vi "ezAFM Practice 1.8.vi"() -> ()   [LabVIEW 2015]
uses:
  <vilib>/userdefined/High Color/IMAQdx.ctl
  D:/LabVIEW for ezAFM/LV-PGC 2019-05a/Special Equipment/ezAFM/NMI Integration Code/ezCommander.dll
  LabVIEW for ezAFM/LV-PGC 2019-05a/Special Equipment/ezAFM/NMI Integration Code/ezCommander.dll
  LabVIEW for ezAFM/LV-PGC 2019-05a/Universal vi's/Global Variables/Globals-EasyAFM.vi
  Helper VI's/Globals.vi
  <vilib>/vision/driver/NI_Vision_Acquisition_Software.lvlib
panel:
  out "Scan Spot Coordinates":dbl[](array[numeric])
  out "Name":string
  out "Sequence Index":dbl
  out "Direction":dbl
  out "Searching":bool
  out "Crosshair Found?":bool
  in  "Search":bool
  out "Total Steps":dbl
  out "Current Steps":dbl
  in  "Camera":enum32{"ezAFM Camera"}(tab)
  out "ezAFM Camera":T1(plugin-control)
  in  "Connection to Scan":string
  in  "Enable Automatic \nRepositioning":bool
  out "Imaging Status":string
  out "Automated Imaging":bool
  in  "Main Menu":T2(tab)
  in  "Navigation Buttons":T3
  in  "Motor Speed":u16(ring)=30000 items=["SLOW"=3300, "MEDIUM"=30000, "FAST"=65000]
  in  "Target Crosshair":string(combo)="00 | 01"
  in  "Current Crosshair":string(combo)="00 | 01"
  in  "MOVE2CROSSHAIR":bool
  in  "THETA":bool
  in  "Angle":dbl
  in  "Step Size":dbl
  in  "Scan Spot":string(combo)
  in  "MOVE2SCANSPOT":bool
  in  "RETRACT":bool
  in  "APPROACH":bool
  in  "SEARCH":bool
  in  "SCAN":bool
  in  "Image Resolution":u16(ring)=256 items=["128"=128, "256"=256, "512"=512, "1024"=1024]
  out "Sequence":string[](array[string])
  out "Connections":string[](array[string])
  in  "Initialize Automated Imaging":bool
  in  "SELECT CONNECTIONS":bool
  in  "ezAFM Default File Path":path=path "D:/ezAFM/Scanned Images"
  in  "Saved Images File Path":path=path "D:/ezAFM/Scanned Images"
  in  "Wafer Type":string(combo)
  in  "Die":string(combo)
  in  "Indicators":enum32{"Indicators"}(tab)
  out "XYZ Motor Position":dbl[](array[numeric]) format="%#_4f"
  out "ezAFM Status":dbl
  out "Approaching":bool
  out "ezAFM Connected":bool
  out "Retracting":bool
  out "Scanning":bool
  out "Tip Approached?":bool
  in  "RESET":bool
  out "XY Position":dbl[](array[numeric])
  in  "QUIT":bool
  # "Use Arrow Keys to manually\nmove the XY Motor"
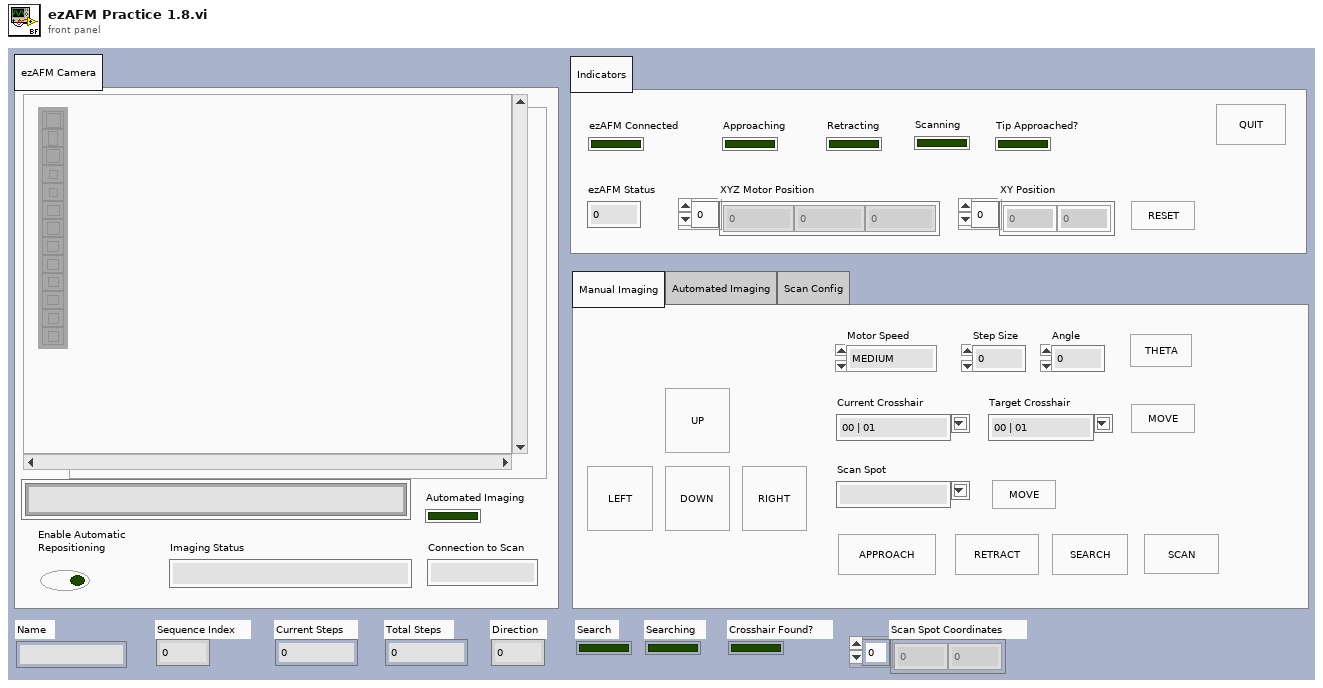
[diagram p1: front panel]
types:
  T1 = typedef "IMAQ Image.ctl" = refnum<image>
  T2 = enum32{"Manual Imaging", "Automated Imaging", "Scan Config"}
  T3 = cluster{"UP":bool, "DOWN":bool, "LEFT":bool, "RIGHT":bool}
  T4 = typedef "IMAQdx.ctl" = refnum<k21>
  T5 = typedef "Image Type" = u32
  T6 = typedef "eventvkey.ctl" = enum16{"ASCII", "Enter", "Return", "Shift", "Ctrl", "Alt", "Cmd", "Opt", "Caps", "NumLock", "Clear", "Break", "Up", "Down", "Left", "Right", "Insert", "Delete", "Home", "End", "PageUp", "PageDown", "Escape", "Help", "Pause", "ScrollLock", "F1", "F2", "F3", "F4", "F5", "F6", "F7", "F8", "F9", "F10", "F11", "F12", "F13", "F14", "F15", "F16", "F17", "F18", "F19", "F20", "F21", "F22", "F23", "F24", "Play", "VolumeUp", "VolumeDown", "Mute", "Two Byte Char"}
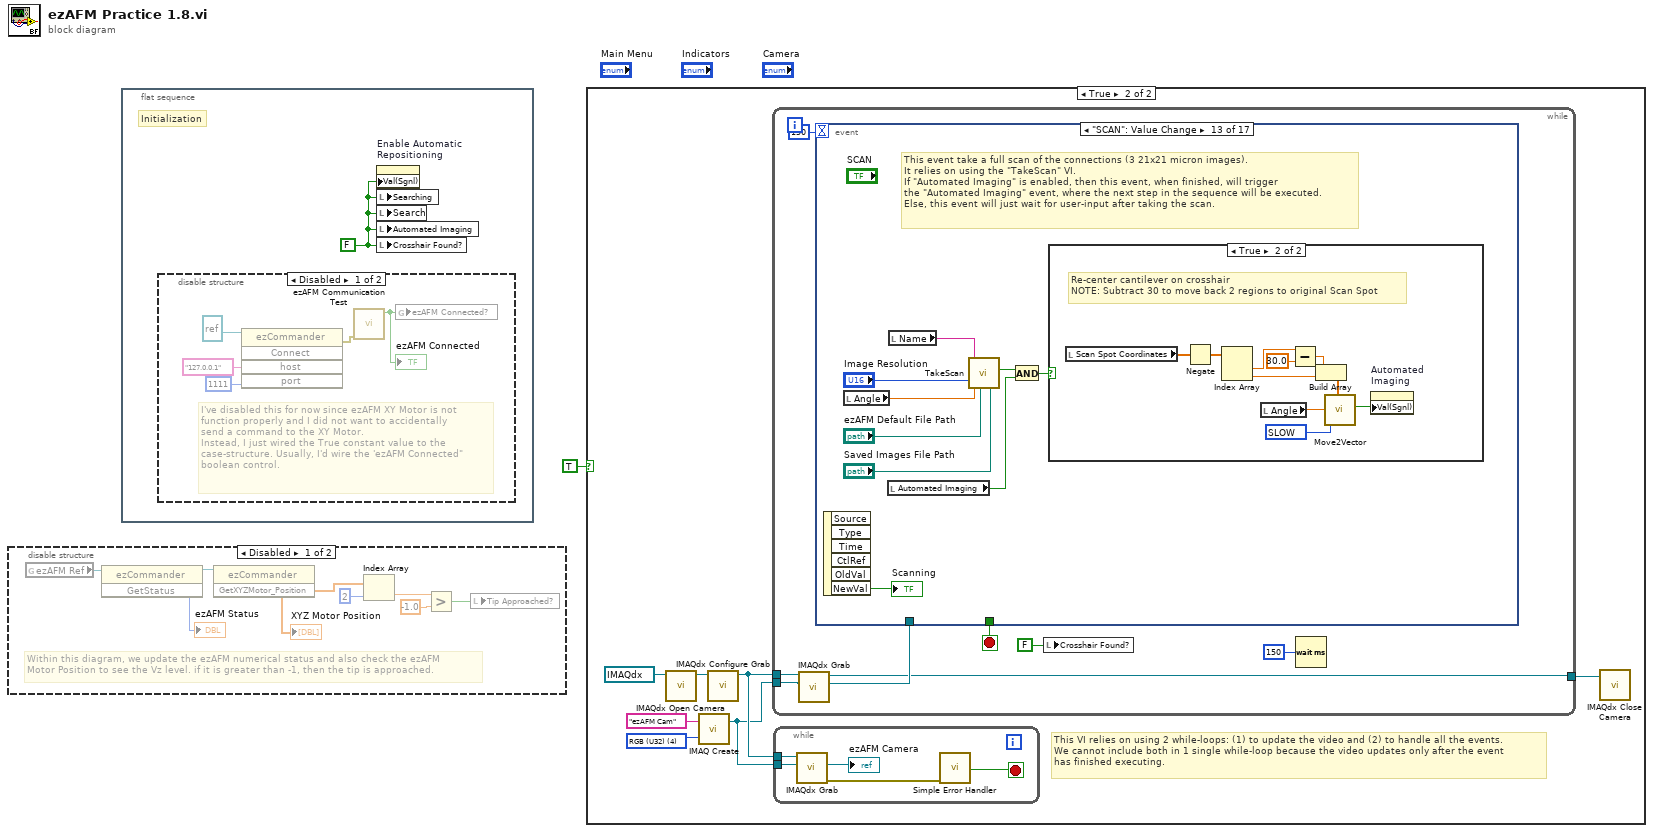
[diagram p0: block diagram]
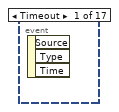
[diagram p5: hidden frame]
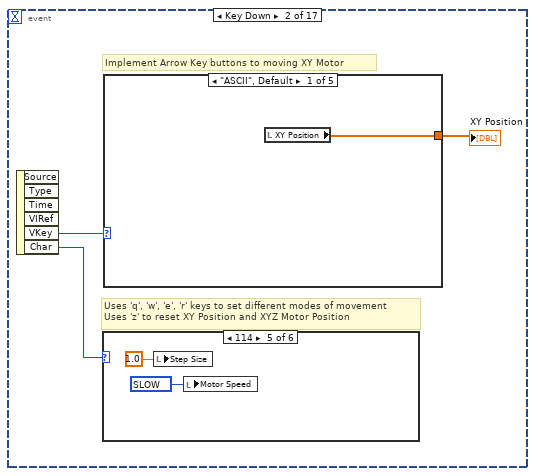
[diagram p6: hidden frame]
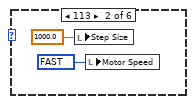
[diagram p8: hidden frame]
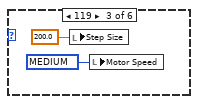
[diagram p9: hidden frame]
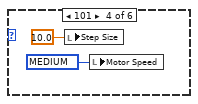
[diagram p10: hidden frame]
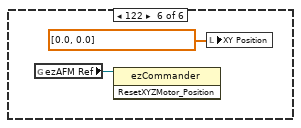
[diagram p11: hidden frame]
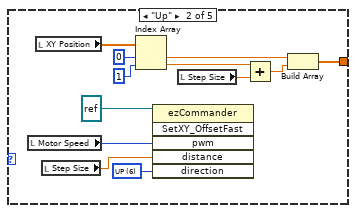
[diagram p12: hidden frame]
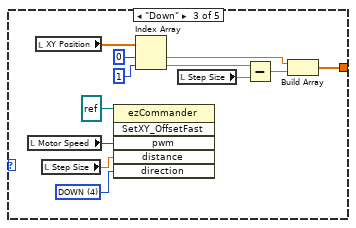
[diagram p13: hidden frame]
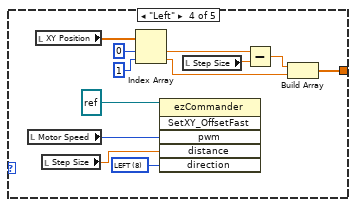
[diagram p14: hidden frame]
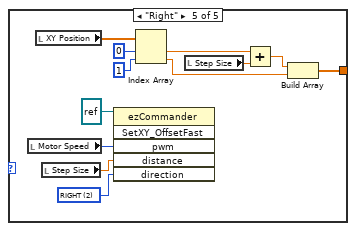
[diagram p15: hidden frame]
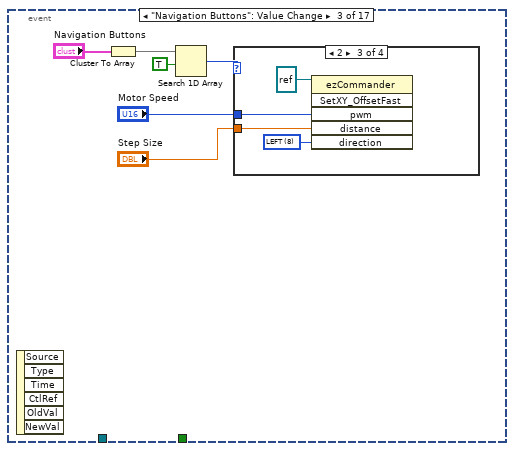
[diagram p16: hidden frame]
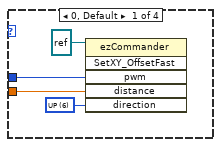
[diagram p17: hidden frame]
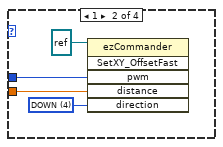
[diagram p18: hidden frame]
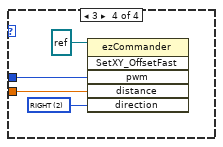
[diagram p19: hidden frame]
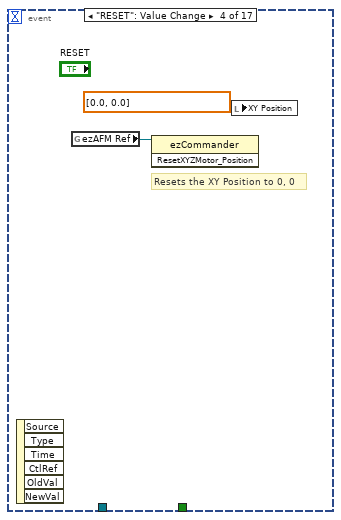
[diagram p20: hidden frame]
diagram:
  n1 = disable-structure shown="Disabled" {
    frame Disabled {
      # "Within this diagram, we update the ezAFM numerical status and also check the ezAFM\nMotor Position to see the Vz level. if it is greater than -1, then the tip is approached."
      n2 = global read "Globals-EasyAFM.vi" "ezAFM Ref"() -> (w7:refnum<k24>)
      n3 = invoke class="ezCommander" method="GetStatus"(reference=w7) -> (reference out=w5:refnum<k24>, "GetStatus"=→"ezAFM Status":i32)  [unwired: 2 in, 1 out]
      n4 = invoke class="ezCommander" method="GetXYZMotor_Position"(reference=w5) -> ("GetXYZMotor_Position"=w9:dbl[])  [unwired: 2 in, 2 out]
      "XYZ Motor Position" <- w9
      n5 = Index Array(array=w9, index=2) -> (element=w4:dbl)
      n6 = Greater?(x=w4, y=-1.0) -> (0:w8:bool)
      n7 = local write "Tip Approached?"(w8) -> ()
    }
    frame Enabled {
    }
  }
  n8 = flat-sequence {
    frame #0 {
      w10 = FALSE ("Automated Imaging")
      # "Initialization"
      n9 = disable-structure shown="Disabled" {
        frame Disabled {
          # "I've disabled this for now since ezAFM XY Motor is not \nfunction properly and I did not want to accidentally\nsend a command to the XY Motor. \nInstead, I just wired the True constant value to the \ncase-structure. Usually, I'd wire the 'ezAFM Connected\"\nboolean control."
          n10 = invoke class="ezCommander" method="Connect"(reference=refnum<k24> refnum ("ezAFM Ref"), "host"="127.0.0.1", "port"=1111) -> (error out=w14:errorcluster)  [unwired: 2 in, 4 out]
          n11 = call "ezAFM Communication Test.vi"("error in"=w14) -> ("ezAFM COM status"=w11:bool)  [unwired: 3 in, 3 out]
          "ezAFM Connected" <- w11
          n12 = global write "Globals.vi" "ezAFM Connected?"(w11) -> ()
        }
        frame Enabled {
        }
      }
      n13 = property on="Enable Automatic \nRepositioning" class="Bool (strict)"("Val(Sgnl)"=w10) -> ()  [unwired: 2 in, 2 out]
      n14 = local write "Searching"(w10) -> ()
      n15 = local write "Search"(w10) -> ()
      n16 = local write "Automated Imaging"(w10) -> ()
      n17 = local write "Crosshair Found?"(w10) -> ()
    }
  }
  n18 = case shown="True" TRUE {
    frame False {
    }
    frame True {
      w19 = T5 4 items=["Grayscale (U8)", "Grayscale (I16)", "Grayscale (SGL)", "Complex (CSG)", "RGB (U32)", "HSL (U32)", "RGB (U64)", "Grayscale (U16)"] ("Image Type")
      # "This VI relies on using 2 while-loops: (1) to update the video and (2) to handle all the events.\nWe cannot include both in 1 single while-loop because the video updates only after the event\nhas finished executing."
      n19 = call <vilib>:"IMAQdx Open Camera.vi"("Session In"=T4 "cam5") -> ("Session Out"=w20:T4)  [unwired: 9 in, 1 out]
      n20 = call "IMAQ Create"("Image Name"="ezAFM Cam", "Image Type"=w19) -> ("New Image"=w17:T1)  [unwired: 3 in, 1 out]
      n21 = call <vilib>:"IMAQdx Configure Grab.vi"("Session In"=w20) -> ("Session Out"=w18:T4)  [unwired: 9 in, 1 out]
      n22 = while {
        tunnel: w18 -> [w33]
        tunnel: w17 -> [w32]
        tunnel: [w30] -> w16
        stop <- w29 stop-if-true
        n23 = call <vilib>:"IMAQdx Grab.vi"("Image In"=w32, "Session In"=w33) -> ("Image Out"=w31:T1, "Session Out"=w30:T4)  [unwired: 2 in, 6 out]
        n24 = event shown="[12] \"SCAN\": Value Change" {
          selector: _ -> [_ _ _ _ _ _ _ _ _ _ _ _ _ _ _ _ _]
          dyn-events: _ -> [_ _ _ _ _ _ _ _ _ _ _ _ _ _ _ _ _]
          timeout: 150 -> [_ _ _ _ _ _ _ _ _ _ _ _ _ _ _ _ _]
          tunnel: [_ _ _ _ _ _ _ _ _ _ _ _ _ _ _ _ "QUIT"] -> w29
          tunnel: w31 -> [_ _ _ _ _ _ _ _ _ _ _ _ _ _ w273 _ _]
          event Timeout {
            n25 = event-data() -> ()  [unwired: 1 in, 3 out]
          }
          event Key Down {
            # "Uses 'q', 'w', 'e', 'r' keys to set different modes of movement\nUses 'z' to reset XY Position and XYZ Motor Position"
            # "Implement Arrow Key buttons to moving XY Motor"
            n26 = event-data() -> ("VKey"=w36:T6, "Char"=w37:i16)  [unwired: 1 in, 4 out]
            n27 = case shown="114" w37 {
              frame 0, Default {
              }
              frame 113 {
                w39 = u16 65000 items=["SLOW"=3300, "MEDIUM"=30000, "FAST"=65000] ("Motor Speed")
                n28 = local write "Step Size"(1000.0 ("Step Size")) -> ()
                n29 = local write "Motor Speed"(w39) -> ()
              }
              frame 119 {
                w41 = u16 30000 items=["SLOW"=3300, "MEDIUM"=30000, "FAST"=65000] ("Motor Speed")
                n30 = local write "Step Size"(200.0 ("Step Size")) -> ()
                n31 = local write "Motor Speed"(w41) -> ()
              }
              frame 101 {
                w43 = u16 30000 items=["SLOW"=3300, "MEDIUM"=30000, "FAST"=65000] ("Motor Speed")
                n32 = local write "Step Size"(10.0 ("Step Size")) -> ()
                n33 = local write "Motor Speed"(w43) -> ()
              }
              frame 114 {
                w45 = u16 3300 items=["SLOW"=3300, "MEDIUM"=30000, "FAST"=65000] ("Motor Speed")
                n34 = local write "Step Size"(1.0 ("Step Size")) -> ()
                n35 = local write "Motor Speed"(w45) -> ()
              }
              frame 122 {
                n36 = global read "Globals-EasyAFM.vi" "ezAFM Ref"() -> (w47:refnum<k24>)
                n37 = invoke class="ezCommander" method="ResetXYZMotor_Position"(reference=w47) -> ()  [unwired: 2 in, 3 out]
                n38 = local write "XY Position"(dbl[] [0.0, 0.0] ("XY Position")) -> ()
              }
            }
            n39 = case shown="\"ASCII\", Default" w36 {
              tunnel: [w49 w51 w62 w74 w86] -> w38
              frame "ASCII", Default {
                n40 = local read "XY Position"() -> (w49:dbl[])
              }
              frame "Up" {
                w60 = u16 6 items=["UP"=6, "DOWN"=4, "LEFT"=8, "RIGHT"=2]
                n41 = local read "Motor Speed"() -> (w59:u16)
                n42 = local read "XY Position"() -> (w57:dbl[])
                n43 = local read "Step Size"() -> (w58:dbl)
                n44 = Index Array(array=w57, index #1=0 ("index"), index #2=1 ("index")) -> (element #1=w53:dbl, element #2=w50:dbl)
                n45 = invoke class="ezCommander" method="SetXY_OffsetFast"(reference=refnum<k24> refnum ("ezAFM Ref"), "pwm"=w59, "distance"=w58, "direction"=w60) -> ()  [unwired: 2 in, 6 out]
                n46 = local read "Step Size"() -> (w54:dbl)
                n47 = Add(x=w50, y=w54) -> (x+y=w52:dbl)
                n48 = Build Array(w53, w52) -> (w51:dbl[])
              }
              frame "Down" {
                w70 = u16 4 items=["UP"=6, "DOWN"=4, "LEFT"=8, "RIGHT"=2]
                n49 = local read "Motor Speed"() -> (w72:u16)
                n50 = local read "XY Position"() -> (w64:dbl[])
                n51 = local read "Step Size"() -> (w71:dbl)
                n52 = invoke class="ezCommander" method="SetXY_OffsetFast"(reference=refnum<k24> refnum ("ezAFM Ref"), "pwm"=w72, "distance"=w71, "direction"=w70) -> ()  [unwired: 2 in, 6 out]
                n53 = Index Array(array=w64, index #1=0 ("index"), index #2=1 ("index")) -> (element #1=w66:dbl, element #2=w67:dbl)
                n54 = local read "Step Size"() -> (w63:dbl)
                n55 = Subtract(x=w67, y=w63) -> (x-y=w65:dbl)
                n56 = Build Array(w66, w65) -> (w62:dbl[])
              }
              frame "Left" {
                w84 = u16 8 items=["UP"=6, "DOWN"=4, "LEFT"=8, "RIGHT"=2]
                n57 = local read "Motor Speed"() -> (w82:u16)
                n58 = local read "XY Position"() -> (w78:dbl[])
                n59 = local read "Step Size"() -> (w83:dbl)
                n60 = Index Array(array=w78, index #1=0 ("index"), index #2=1 ("index")) -> (element #1=w77:dbl, element #2=w75:dbl)
                n61 = invoke class="ezCommander" method="SetXY_OffsetFast"(reference=refnum<k24> refnum ("ezAFM Ref"), "pwm"=w82, "distance"=w83, "direction"=w84) -> ()  [unwired: 2 in, 6 out]
                n62 = local read "Step Size"() -> (w79:dbl)
                n63 = Subtract(x=w77, y=w79) -> (x-y=w76:dbl)
                n64 = Build Array(w76, w75) -> (w74:dbl[])
              }
              frame "Right" {
                w96 = u16 2 items=["UP"=6, "DOWN"=4, "LEFT"=8, "RIGHT"=2]
                n65 = local read "Motor Speed"() -> (w95:u16)
                n66 = local read "XY Position"() -> (w91:dbl[])
                n67 = local read "Step Size"() -> (w94:dbl)
                n68 = invoke class="ezCommander" method="SetXY_OffsetFast"(reference=refnum<k24> refnum ("ezAFM Ref"), "pwm"=w95, "distance"=w94, "direction"=w96) -> ()  [unwired: 2 in, 6 out]
                n69 = Index Array(array=w91, index #1=0 ("index"), index #2=1 ("index")) -> (element #1=w89:dbl, element #2=w87:dbl)
                n70 = local read "Step Size"() -> (w90:dbl)
                n71 = Add(x=w89, y=w90) -> (x+y=w88:dbl)
                n72 = Build Array(w88, w87) -> (w86:dbl[])
              }
            }
            "XY Position" <- w38
          }
          event "Navigation Buttons": Value Change {
            n73 = event-data() -> ()  [unwired: 1 in, 6 out]
            n74 = Cluster To Array(cluster="Navigation Buttons") -> (array=w102:bool[])
            n75 = Search 1D Array(1D array=w102, element=TRUE) -> (index of element=w100:i32)  [unwired: 1 in]
            n76 = case shown="2" w100 {
              tunnel: "Step Size" -> [w104 w109 w113 w117]
              tunnel: "Motor Speed" -> [w105 w108 w112 w116]
              frame 0, Default {
                w106 = u16 6 items=["UP"=6, "DOWN"=4, "LEFT"=8, "RIGHT"=2]
                n77 = invoke class="ezCommander" method="SetXY_OffsetFast"(reference=refnum<k24> refnum ("ezAFM Ref"), "pwm"=w105, "distance"=w104, "direction"=w106) -> ()  [unwired: 2 in, 6 out]
              }
              frame 1 {
                w110 = u16 4 items=["UP"=6, "DOWN"=4, "LEFT"=8, "RIGHT"=2]
                n78 = invoke class="ezCommander" method="SetXY_OffsetFast"(reference=refnum<k24> refnum ("ezAFM Ref"), "pwm"=w108, "distance"=w109, "direction"=w110) -> ()  [unwired: 2 in, 6 out]
              }
              frame 2 {
                w114 = u16 8 items=["UP"=6, "DOWN"=4, "LEFT"=8, "RIGHT"=2]
                n79 = invoke class="ezCommander" method="SetXY_OffsetFast"(reference=refnum<k24> refnum ("ezAFM Ref"), "pwm"=w112, "distance"=w113, "direction"=w114) -> ()  [unwired: 2 in, 6 out]
              }
              frame 3 {
                w118 = u16 2 items=["UP"=6, "DOWN"=4, "LEFT"=8, "RIGHT"=2]
                n80 = invoke class="ezCommander" method="SetXY_OffsetFast"(reference=refnum<k24> refnum ("ezAFM Ref"), "pwm"=w116, "distance"=w117, "direction"=w118) -> ()  [unwired: 2 in, 6 out]
              }
            }
          }
          event "RESET": Value Change {
            # "Resets the XY Position to 0, 0"
            n81 = event-data() -> ()  [unwired: 1 in, 6 out]
            n82 = global read "Globals-EasyAFM.vi" "ezAFM Ref"() -> (w120:refnum<k24>)
            n83 = invoke class="ezCommander" method="ResetXYZMotor_Position"(reference=w120) -> ()  [unwired: 2 in, 3 out]
            n84 = local write "XY Position"(dbl[] [0.0, 0.0] ("XY Position")) -> ()
          }
          event "THETA": Value Change {
            # "NOTE: 9/17/2019: This feature does not work reliably because XY Position is a simple record of horizontal\nand vertical movements without accounting for Motor Speed. Different Motor Speeds lead to different\nerror and physical distance values.\nI've noticed that using any generic angle measurement tool such as Windows Snip and entering the estimated angle\ninto the control value works sufficiently."
            # "Takes the absolute value of the XY Position and computes the magnitude of the angle.\nThen based on the sign of the X and Y position, we change the sign of the angle\nIf both signs are the same, then the angle should be negative (clockwise rotated by theta)\nElse if both signs are different, then the angle should be positive (counter-clockwise rotated)"
            n85 = event-data() -> ()  [unwired: 1 in, 6 out]
            n86 = local read "XY Position"() -> (w135:dbl[])
            n87 = Absolute Value(x=w135) -> (abs(x)=w136:dbl[])
            n88 = Index Array(array=w135) -> (element #1=w129:dbl, element #2=w128:dbl)  [unwired: 2 in]
            n89 = Index Array(array=w136, index #1=1 ("index"), index #2=0 ("index")) -> (element #1=w132:dbl, element #2=w131:dbl)
            n90 = Re/Im To Complex(1:w131, 2:w132) -> (0:w130:cdb)
            n91 = Sign(1:w129) -> (0:w127:dbl)
            n92 = Sign(1:w128) -> (0:w126:dbl)
            n93 = Complex To Polar(r * e^(i*theta)=w130) -> (theta=w124:dbl)  [unwired: 1 out]
            n94 = Equal?(x=w127, y=w126) -> (x = y?=w125:bool)
            n95 = case shown="True" w125 {
              tunnel: w124 -> [w137 w139]
              tunnel: [w137 w138] -> w123
              frame False {
              }
              frame True {
                n96 = Negate(x=w139) -> (-x=w138:dbl)
              }
            }
            n97 = expression code="(x/pi)*180.0" "radians to degrees"(w123) -> (w122:dbl)
            n98 = local write "Angle"(w122) -> ()
          }
          event "APPROACH", "RETRACT": Value Change {
            n99 = event-data() -> ()  [unwired: 1 in, 6 out]
            n100 = case shown="True" "APPROACH" {
              selector: "APPROACH" -> [_ w148]
              frame False {
              }
              frame True {
                n101 = call "AutoLand&Approach.vi"("Autoland?"=w148, "Step-Approach?"=FALSE) -> ("Finished?"=w147:bool)
                "Tip Approached?" <- w147
                n102 = Not(x=w147) -> (.not. x?=w149:bool)
                n103 = local write "Approaching"(w149) -> ()
                "Approaching" <- w148
              }
            }
            n104 = case shown="True" "RETRACT" {
              selector: "RETRACT" -> [_ w142]
              frame False {
              }
              frame True {
                n105 = call "Retract.vi"("Number of Cycles"=10, "Retracting?"=w142) -> ("Finished?"=w144:bool)
                n106 = Not(x=w144) -> (.not. x?=w143:bool)
                n107 = local write "Tip Approached?"(w143) -> ()
                n108 = local write "Retracting"(w143) -> ()
                "Retracting" <- w142
              }
            }
          }
          event "SELECT CONNECTIONS": Value Change {
            # "This event calls the \"SelectConnections\" VI which is just my helper VI that lets the user click which connections\nthey're interested in.  \nThe next version \"ezAFM Practice 1.9\" VI will include a rough draft of my attempt to replace \nthis event by integrating the \"ShowAllConnections\" VI along with the \"SimpleMap\" VI."
            n109 = event-data() -> ()  [unwired: 1 in, 6 out]
            n110 = case shown="True" "SELECT CONNECTIONS" {
              frame False {
              }
              frame True {
                n111 = call "SelectConnections.vi"() -> ("Selected Connections"=→"Connections":string[])  [unwired: 1 in]
              }
            }
          }
          event "Initialize Automated Imaging": Value Change {
            # "This event initializes the parameters for \"Automated Imaging\".\nIt uses the \"BuildSeqeuence' VI to create a string array of movements.\nAlso, this event enables \"Automatic Repositioning\" to find the crosshair."
            n112 = event-data() -> ()  [unwired: 1 in, 6 out]
            n113 = local read "Connections"() -> (w156:string[])
            n114 = call "BuildSequence.vi"("Connections"=w156) -> ("Sequence"=w154:string[])
            "Sequence" <- w154
            n115 = Array Size(array=w154) -> (size(s)=w153:i32)
            n116 = Greater Than 0?(x=w153) -> (x > 0?=w152:bool)
            n117 = local write "Enable Automatic \nRepositioning"(w152) -> ()
            n118 = local write "Automated Imaging"(w152) -> ()
            n119 = property on="Automated Imaging" class="Bool (strict)"("Val(Sgnl)"=w152) -> ()  [unwired: 2 in, 2 out]
            "Sequence Index" <- -1.0 ("Index")
          }
          event "Automated Imaging": Value Change {
            # "This event is sort of the \"main\" event running the Automated Imaging. It relies on other events such as\n\"MOVE2SCANSPOT\" and \"MOVE2CROSSHAIR\".\nWe test substrings within each step in the Sequence to judge whether to execute Coarse or Fine\nmovement commads."
            # "Iterate through the Sequence array"
            n120 = event-data() -> ()  [unwired: 1 in, 6 out]
            n121 = local read "Sequence Index"() -> (w160:dbl)
            n122 = local read "Sequence"() -> (w158:string[])
            n123 = Increment(x=w160) -> (x+1=w159:dbl)
            n124 = local write "Sequence Index"(w159) -> ()
            n125 = Index Array(array=w158, index=w159) -> (element=w157:string)
            "Imaging Status" <- w157
            n126 = Search/Split String(string=w157, search string/char (-)="Scan Spot") -> (offset of match=w163:i32)  [unwired: 1 in, 2 out]
            n127 = Search/Split String(string=w157, search string/char (-)="Crosshairs") -> (offset of match=w164:i32)  [unwired: 1 in, 2 out]
            n128 = Greater Or Equal To 0?(x=w163) -> (x >= 0?=w162:bool)
            n129 = Greater Or Equal To 0?(x=w164) -> (x >= 0?=w161:bool)
            n130 = case shown="True" w161 {
              tunnel: w157 -> [_ w174]
              frame False {
              }
              frame True {
                n131 = String Subset(string=w174, offset (0)=21, length (rest)=7 ("length (rest)")) -> (substring=w168:string)
                n132 = String Subset(string=w174, offset (0)=10, length (rest)=7 ("length (rest)")) -> (substring=w169:string)
                n133 = String Length(string=w169) -> (length=w170:i32)
                n134 = String Length(string=w168) -> (length=w171:i32)
                n135 = local write "Current Crosshair"(w169) -> ()
                n136 = local write "Target Crosshair"(w168) -> ()
                n137 = Greater Than 0?(x=w170) -> (x > 0?=w172:bool)
                n138 = Greater Than 0?(x=w171) -> (x > 0?=w173:bool)
                n139 = And(x=w172, y=w173) -> (x .and. y?=w167:bool)
                n140 = property on="MOVE2CROSSHAIR" class="Bool (strict)"("Val(Sgnl)"=w167) -> ()  [unwired: 2 in, 2 out]
              }
            }
            n141 = case shown="True" w162 {
              tunnel: w157 -> [_ w187]
              tunnel: w157 -> [_ w179]
              frame False {
              }
              frame True {
                n142 = String Subset(string=w187, offset (0)=18, length (rest)=2 ("length (rest)")) -> (substring=w182:string)
                n143 = String Subset(string=w179, offset (0)=25) -> (substring=w181:string)  [unwired: 1 in]
                n144 = local write "Scan Spot"(w182) -> ()
                n145 = local write "Connection to Scan"(w181) -> ()
                n146 = String Length(string=w182) -> (length=w183:i32)
                n147 = String Length(string=w181) -> (length=w184:i32)
                n148 = Greater Than 0?(x=w183) -> (x > 0?=w185:bool)
                n149 = Greater Than 0?(x=w184) -> (x > 0?=w186:bool)
                n150 = And(x=w185, y=w186) -> (x .and. y?=w180:bool)
                n151 = property on="MOVE2SCANSPOT" class="Bool (strict)"("Val(Sgnl)"=w180) -> ()  [unwired: 2 in, 2 out]
              }
            }
          }
          event "MOVE2CROSSHAIR": Value Change {
            w196 = u16 65000 items=["SLOW"=3300, "MEDIUM"=30000, "FAST"=65000] ("Motor Speed")
            # "After moving to the Target Crosshair, this event triggers the \"Search\" event \ndepending on if 'Enable Automatic Repositioning\" is true.\nNOTE: We would set \"Enable Automatic Repositioning\" to be true in the \"Initialize Automated Imaging\" event."
            # "This event addresses Coarse Navigation.\nIt uses the \"GetCrosshairVector\" VI to generate the \nXY Vector representing the relative distance between the \n\"Current\" and \"Target\" Crosshair pertaining to a pair of devices"
            n152 = event-data() -> ()  [unwired: 1 in, 6 out]
            n153 = call "GetCrosshairVector.vi"("Target Crosshair"="Target Crosshair", "Current Crosshair"="Current Crosshair") -> ("XY Vector"=w191:dbl[])  [unwired: 9 in]
            n154 = local read "Angle"() -> (w195:dbl)
            n155 = call "Move2Vector.vi"("Motor Speed"=w196, "Angle"=w195, "XY Vector"=w191) -> ("Finished?"=w194:bool)  [unwired: 8 in]
            n156 = case shown="True" w194 {
              frame False {
              }
              frame True {
                n157 = local read "Enable Automatic \nRepositioning"() -> (w199:bool)
                n158 = local read "Target Crosshair"() -> (w198:string)
                n159 = local write "MOVE2CROSSHAIR"(FALSE) -> ()
                n160 = local write "Current Crosshair"(w198) -> ()
                n161 = case shown="True" w199 {
                  selector: w199 -> [_ w200]
                  frame False {
                  }
                  frame True {
                    n162 = property on="Search" class="Bool (strict)"("Val(Sgnl)"=w200) -> ()  [unwired: 2 in, 2 out]
                  }
                }
              }
            }
          }
          event "MOVE2SCANSPOT": Value Change {
            w206 = u16 3300 items=["SLOW"=3300, "MEDIUM"=30000, "FAST"=65000] ("Motor Speed")
            # "This event addresses Fine Navigation.\nIt refers to my other helper VI, called \"GetScanSpot\", to obtain the scan spot \ncoordinates for A0, B0, A1, B1. \nIf \"Automated Imaging\" is enabled, then this event, when finished, triggers the \n\"SCAN\" event. \nElse, this will just wait for user-input after moving to the scan spot."
            n163 = event-data() -> ()  [unwired: 1 in, 6 out]
            n164 = for {
              tunnel: string[] ["X edge even", "X edge odd", "Y edge efgh", "Y edge abcde"] -> [w238] mode=indexing
              tunnel: [w237] -> w209 mode=indexing
              n165 = Current VI's Path() -> (path=w245:path)
              n166 = Strip Path(path=w245) -> (stripped path=w244:path)  [unwired: 1 out]
              n167 = Build Path(base path=w244, name or relative path="GetScanSpot.vi") -> (appended path=w242:path)
              n168 = Open VI Reference(vi path=w242) -> (vi reference=w241:refnum<vi>)  [unwired: 5 in, 1 out]
              n169 = invoke class="VI" method="Ctrl Val.Get"(reference=w241, "Control Name"=w238) -> ("Get Control Value Variant"=w240:variant)  [unwired: 2 in, 3 out]
              n170 = Variant To Data(type=0.0, Variant=w240) -> (data=w237:dbl)  [unwired: 1 in, 1 out]
            }
            n171 = case shown="\"B0\"" "Scan Spot" {
              tunnel: w209 -> [_ w217 w219 w225 w231]
              tunnel: [w211 w212 w218 w224 w230] -> w210
              tunnel: [w211 w212 w218 w224 w230] -> w201
              frame Default {
                w211 = dbl[] [0.0, 0.0] ("XY Vector")
              }
              frame "A0" {
                n172 = Index Array(array=w217, index #1=0 ("index"), index #2=3 ("index")) -> (element #1=w214:dbl, element #2=w213:dbl)
                n173 = Build Array(w214, w213) -> (w212:dbl[])
              }
              frame "B0" {
                n174 = Index Array(array=w219, index #1=0 ("index"), index #2=2 ("index")) -> (element #1=w221:dbl, element #2=w220:dbl)
                n175 = Build Array(w221, w220) -> (w218:dbl[])
              }
              frame "A1" {
                n176 = Index Array(array=w225, index #1=1 ("index"), index #2=3 ("index")) -> (element #1=w227:dbl, element #2=w226:dbl)
                n177 = Build Array(w227, w226) -> (w224:dbl[])
              }
              frame "B1" {
                n178 = Index Array(array=w231, index #1=1 ("index"), index #2=2 ("index")) -> (element #1=w233:dbl, element #2=w232:dbl)
                n179 = Build Array(w233, w232) -> (w230:dbl[])
              }
            }
            "Scan Spot Coordinates" <- w201
            n180 = local read "Angle"() -> (w207:dbl)
            n181 = local read "Automated Imaging"() -> (w205:bool)
            n182 = call "Move2Vector.vi"("Motor Speed"=w206, "Angle"=w207, "XY Vector"=w210) -> ("Finished?"=w204:bool)  [unwired: 8 in]
            n183 = And(x=w204, y=w205) -> (x .and. y?=w203:bool)
            n184 = case shown="True" w203 {
              selector: w203 -> [_ w236]
              frame False {
              }
              frame True {
                n185 = property on="SCAN" class="Bool (strict)"("Val(Sgnl)"=w236) -> ()  [unwired: 2 in, 2 out]
              }
            }
          }
          event "Connection to Scan": Value Change {
            # "This event simply updates the \"Name\" indicator for when we save the image files after\ntaking a scan. (\"Name\" is used as a parameter in the \"TakeScan\" VI)"
            n186 = event-data() -> ()  [unwired: 1 in, 6 out]
            n187 = Concatenate Strings("Wafer Type", "-" ("string"), "Die", "Connection to Scan") -> (→"Name":string)
          }
          event "SCAN": Value Change {
            # "This event take a full scan of the connections (3 21x21 micron images).\nIt relies on using the \"TakeScan\" VI.\nIf \"Automated Imaging\" is enabled, then this event, when finished, will trigger\nthe \"Automated Imaging\" event, where the next step in the sequence will be executed.\nElse, this event will just wait for user-input after taking the scan."
            n188 = event-data() -> ("NewVal"=→"Scanning":bool)  [unwired: 1 in, 5 out]
            n189 = local read "Angle"() -> (w257:dbl)
            n190 = local read "Automated Imaging"() -> (w252:bool)
            n191 = local read "Name"() -> (w259:string)
            n192 = call "TakeScan.vi"("Target File Path"="Saved Images File Path", "ezAFM Default Path"="ezAFM Default File Path", "Angle"=w257, "Image Resolution"="Image Resolution", "Name"=w259) -> ("Finished?"=w253:bool)  [unwired: 6 in]
            n193 = And(x=w253, y=w252) -> (x .and. y?=w251:bool)
            n194 = case shown="True" w251 {
              frame False {
              }
              frame True {
                w267 = u16 3300 items=["SLOW"=3300, "MEDIUM"=30000, "FAST"=65000] ("Motor Speed")
                # "Re-center cantilever on crosshair\nNOTE: Subtract 30 to move back 2 regions to original Scan Spot"
                n195 = local read "Scan Spot Coordinates"() -> (w260:dbl[])
                n196 = Negate(x=w260) -> (-x=w261:dbl[])
                n197 = Index Array(array=w261) -> (element #1=w263:dbl, element #2=w264:dbl)  [unwired: 2 in]
                n198 = local read "Angle"() -> (w268:dbl)
                n199 = Subtract(x=w263, y=30.0) -> (x-y=w265:dbl)
                n200 = Build Array(w265, w264) -> (w266:dbl[])
                n201 = call "Move2Vector.vi"("Motor Speed"=w267, "Angle"=w268, "XY Vector"=w266) -> ("Finished?"=w269:bool)  [unwired: 8 in]
                n202 = property on="Automated\nImaging" class="Bool (strict)"("Val(Sgnl)"=w269) -> ()  [unwired: 2 in, 2 out]
              }
            }
          }
          event "Enable Automatic \nRepositioning": Value Change {
            w270 = u16 6 items=["UP"=6, "DOWN"=4, "LEFT"=8, "RIGHT"=2]
            # "This event initializes the parameters involved for my \"Automatic Repositioning\", \nalgorithm which includes 3 events; this one, \"Search\", and \"Searching\""
            n203 = event-data() -> ()  [unwired: 1 in, 6 out]
            "Total Steps" <- 1.0 ("Total Distance")
            "Current Steps" <- 0.0 ("Current Steps")
            "Direction" <- w270
          }
          event "SEARCH", "Search": Value Change {
            # "This event uses the \"IdentifyCrosshair\" VI to obtain the coordinates to the \ncenter of the crosshairs, which are then are passed into the \"Move2Vector\" VI.\n\nIf \"Automatic Repositioning\" is enabled, then, in the case of no crosshair found,\nthis event triggers the \"Searching\" event.\nElse, this event will just wait for user-input after attempting to identify the crosshair."
            n204 = event-data() -> ("NewVal"=w274:bool)  [unwired: 1 in, 5 out]
            n205 = while {
              tunnel: w273 -> [w283]
              tunnel: [w279] -> w275
              tunnel: [w282] -> w276
              i -> [w280]
              stop <- w277 stop-if-true
              n206 = Greater?(x=w280, y=5.0) -> (0:w278:bool)
              n207 = call "IdentifyCrosshair.vi"("ezAFM Camera"=w283) -> ("Delta"=w282:dbl[], "Found?"=w279:bool)
              n208 = Or(x=w278, y=w279) -> (x .or. y?=w277:bool)
            }
            "Crosshair Found?" <- w275
            n209 = local write "Searching"(w274) -> ()
            n210 = case shown="False" w275 {
              tunnel: w276 -> [_ w294]
              frame False {
                n211 = local read "Enable Automatic \nRepositioning"() -> (w285:bool)
                n212 = local write "Searching"(FALSE ("Searching")) -> ()
                n213 = case shown="True" w285 {
                  frame False {
                  }
                  frame True {
                    n214 = property on="Searching" class="Bool (strict)"("Val(Sgnl)"=TRUE ("Value (Signaling)")) -> ()  [unwired: 2 in, 2 out]
                  }
                }
              }
              frame True {
                w292 = FALSE ("SEARCH")
                w293 = u16 3300 items=["SLOW"=3300, "MEDIUM"=30000, "FAST"=65000] ("Motor Speed")
                n215 = local write "Search"(w292) -> ()
                n216 = local write "Searching"(w292) -> ()
                n217 = call "Move2Vector.vi"("Motor Speed"=w293, "Angle"=0.0, "XY Vector"=w294) -> ("Finished?"=w288:bool)  [unwired: 8 in]
                n218 = local read "Automated Imaging"() -> (w287:bool)
                n219 = property on="Enable Automatic \nRepositioning" class="Bool (strict)"("Val(Sgnl)"=TRUE ("Value (Signaling)")) -> ()  [unwired: 2 in, 2 out]
                n220 = And(x=w288, y=w287) -> (x .and. y?=w289:bool)
                n221 = case shown="True" w289 {
                  selector: w289 -> [_ w295]
                  frame False {
                  }
                  frame True {
                    n222 = property on="Automated Imaging" class="Bool (strict)"("Val(Sgnl)"=w295) -> ()  [unwired: 2 in, 2 out]
                  }
                }
              }
            }
          }
          event "Searching": Value Change {
            # "At the end of the movement, this event triggers the \"Search\" event to atttempt\nto identify the crosshair."
            # "This event takes in the parameters for \"Automatic Repositioning and sends commands to the\nXY Motor to move in a certain direction. \nThe overall pattern of movement resembles a square spiral."
            n223 = event-data() -> ()  [unwired: 1 in, 6 out]
            n224 = local read "Total Steps"() -> (w298:dbl)
            n225 = local read "Current Steps"() -> (w299:dbl)
            n226 = local read "Direction"() -> (w300:dbl)
            n227 = Equal?(x=w298, y=w299) -> (x = y?=w301:bool)
            n228 = case shown="False" w301 {
              tunnel: w299 -> [w306 _]
              tunnel: w300 -> [w307 w316]
              tunnel: w298 -> [w302 w312]
              tunnel: [TRUE ("Value (Signaling)") TRUE ("Value (Signaling)")] -> w297
              tunnel: [w302 w311] -> w296
              frame False {
                w308 = u16 65000 items=["SLOW"=3300, "MEDIUM"=30000, "FAST"=65000] ("Motor Speed")
                n229 = Increment(x=w306) -> (x+1=w305:dbl)
                n230 = local write "Current Steps"(w305) -> ()
                n231 = invoke class="ezCommander" method="SetXY_OffsetFast"(reference=refnum<k24> refnum ("ezAFM Ref"), "pwm"=w308, "distance"=20.0, "direction"=w307) -> ()  [unwired: 2 in, 6 out]
                n232 = Wait (ms)(milliseconds to wait=u32 1000) -> ()  [unwired: 1 out]
              }
              frame True {
                n233 = case shown="6" w316 {
                  tunnel: [u16 0 w319 w320 w321 w322] -> w315
                  frame Default {
                  }
                  frame 6 {
                    w319 = u16 2 items=["UP"=6, "DOWN"=4, "LEFT"=8, "RIGHT"=2]
                  }
                  frame 4 {
                    w320 = u16 8 items=["UP"=6, "DOWN"=4, "LEFT"=8, "RIGHT"=2]
                  }
                  frame 8 {
                    w321 = u16 6 items=["UP"=6, "DOWN"=4, "LEFT"=8, "RIGHT"=2]
                  }
                  frame 2 {
                    w322 = u16 4 items=["UP"=6, "DOWN"=4, "LEFT"=8, "RIGHT"=2]
                  }
                }
                n234 = local write "Current Steps"(0.0 ("Current Steps")) -> ()
                n235 = local write "Direction"(w315) -> ()
                n236 = Increment(x=w312) -> (x+1=w311:dbl)
                n237 = Wait (ms)(milliseconds to wait=u32 1000) -> ()  [unwired: 1 out]
              }
            }
            n238 = property on="Search" class="Bool (strict)"("Val(Sgnl)"=w297) -> ()  [unwired: 2 in, 2 out]
            n239 = local write "Total Steps"(w296) -> ()
          }
          event "QUIT": Value Change {
            w324 = FALSE ("ezAFM Connected?")
            n240 = event-data() -> ()  [unwired: 1 in, 6 out]
            n241 = global write "Globals.vi" "ezAFM Connected?"(w324) -> ()
            n242 = local write "ezAFM Connected"(w324) -> ()
          }
        }
        n243 = local write "Crosshair Found?"(FALSE ("Scan")) -> ()
        n244 = Wait (ms)(milliseconds to wait=u32 150) -> ()  [unwired: 1 out]
      }
      n245 = while {
        tunnel: w18 -> [w27]
        tunnel: w17 -> [w26]
        stop <- w23 stop-if-true
        n246 = call <vilib>:"IMAQdx Grab.vi"("Image In"=w26, "Session In"=w27) -> ("error out"=w24:errorcluster, "Image Out"=→"ezAFM Camera":T1)  [unwired: 2 in, 6 out]
        n247 = call <vilib>:"Simple Error Handler.vi"("error in (no error)"=w24) -> ("error?"=w23:bool)  [unwired: 4 in, 4 out]
      }
      n248 = call <vilib>:"IMAQdx Close Camera.vi"("Session In"=w16) -> ()  [unwired: 10 in, 1 out]
    }
  }
